vi "Pre Launch Init.vi"(11 "DAQmx Delay Line in":refnum<class "DAQmx Delay Line.lvclass">) -> (0 "error out":errorcluster, 3 "DAQmx Delay Line out":refnum<class "DAQmx Delay Line.lvclass">)   [LabVIEW 2016, in "Delay Line.lvlib" / "DAQmx Delay Line.lvclass"]
doc: "(<B>Filename</B>: Actor Framework.lvlib:Actor.lvclass:Pre Launch Init.vi)\n\nDefines behavior that occurs after the Launch Nested Actor method is invoked but before the actor's Actor Core method begins running.\n\nBy default, this method does nothing. A descendant class may override it to define behavior."
uses:
  DAQmx Delay Line.lvclass
  Abstract Delay Line/Abstract Delay Line.lvclass
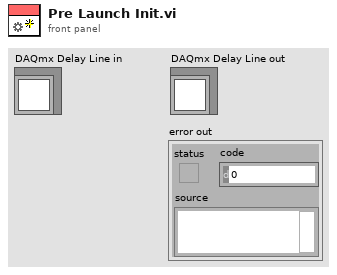
[diagram p1: front panel]
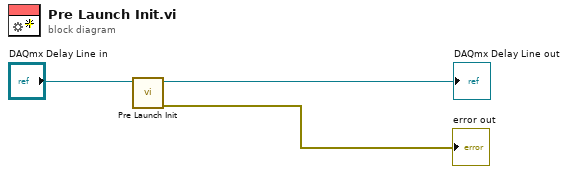
[diagram p0: block diagram]
diagram:
  n1 = call-parent "Pre Launch Init.vi"("Actor in"="DAQmx Delay Line in") -> ("error out"=→"error out":errorcluster, "Actor out"=→"DAQmx Delay Line out":refnum<class "DAQmx Delay Line.lvclass">)  [unwired: 9 in]
